vi "NotAnOccurrence.vi"(1 "occurrence refnum":refnum<k4>) -> (0 "not an occurrence?":bool)   [LabVIEW 2019, in "_ChannelSupport.lvlib"]
uses:
  _ChannelSupport.lvlib
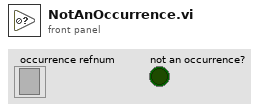
[diagram p1: front panel]
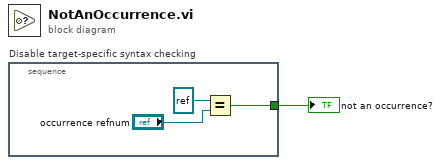
[diagram p0: block diagram]
diagram:
  n1 = stacked-sequence "Disable target-specific syntax checking" {
    tunnel: [w2] -> w1
    frame #0 {
      n2 = Equal?(x=refnum<k4> refnum, y="occurrence refnum") -> (x = y?=w2:bool)
    }
  }
  "not an occurrence?" <- w1
